vi "Scatter-Gather Read Iterator.vi"(8 "error in (no error)":errorcluster, 9 "Iterations (1000)":i32=110, 10 "Channel Count":i32, 11 "GE 5565PIORC in":refnum<class "GE 5565PIORC.lvclass">) -> (0 "error out":errorcluster, 1 "Histogram Graph":T1(graph), 2 "Metrics":T2 {"Transfer Rate" format="%.2pB/s"; "Duration Std. Dev." format="%.0f µs"; "Duration Average" format="%.0f µs"}, 3 "GE 5565PIORC out":refnum<class "GE 5565PIORC.lvclass">)   [LabVIEW 2016]
uses:
  Source/GE 5565PIORC/GE 5565PIORC.lvclass
  Controls/Throughput Metrics.ctl
  Source/GE 5565PIORC/GE 5565PIORC.lvclass/GE 5565PIORC.ctl
  Source/GE 5565PIORC/VIs/DMA/DMA.Start Transfer.vi
  Source/GE 5565PIORC/VIs/DMA/DMA.Wait for Done Interrupt Event.vi
  Source/GE 5565PIORC/VIs/Interrupts/Discard PXI Interrupt Events.vi
  Source/GE 5565PIORC/VIs/DMA/DMA.Configure.vi
  Source/GE 5565PIORC/VIs/Registers/Local Configuration.DMACSR0.DMA Start.Set.vi
  Source/GE 5565PIORC/VIs/Interrupts/Wait for PXI Interrupt Events.vi
  Source/GE 5565PIORC/VIs/Registers/Local Configuration.DMACSR0.DMA Clear Interrupt.Set.vi
  <vilib>/Utility/error.llb/Clear Errors.vi
  Source/GE 5565PIORC/VIs/Registers/Local Configuration.PCI Address.Set.vi
  Source/GE 5565PIORC/VIs/Registers/Local Configuration.DMADPR0.First Descriptor Address.Set.vi
  Source/GE 5565PIORC/VIs/DMA/DMA.Scatter-Gather.Link Block Descriptors.vi
  Source/GE 5565PIORC/VIs/DMA/DMA.Scatter-Gather.Commit Blocks.vi
  Source/GE 5565PIORC/VIs/Registers/Local Configuration.Local Address.Set.vi
  Source/GE 5565PIORC/VIs/Registers/Local Configuration.Transfer Size.Set.vi
  Source/GE 5565PIORC/VIs/Registers/Local Configuration.DMADPR0.Transfer Direction.Set.vi
  Source/GE 5565PIORC/VIs/Registers/Local Configuration.DMAMODE0.Scatter-Gather Enable.Set.vi
  Source/GE 5565PIORC/VIs/Binary Operations/Set Bits.vi
  Source/GE 5565PIORC/VIs/Binary Operations/Set Bits U32.vi
  Source/GE 5565PIORC/VIs/Registers/Local Configuration.Get Register Offset.vi
  Source/GE 5565PIORC/VIs/Binary Operations/Get Bits.vi
  Source/GE 5565PIORC/VIs/Binary Operations/Get Bits U32.vi
  Source/GE 5565PIORC/VIs/Block Operations/Allocate Multiple Blocks.vi
  Source/GE 5565PIORC/VIs/DMA/DMA.Create Transfer (Multiple Blocks).vi
  Source/GE 5565PIORC/VIs/DMA/DMA.Transfer Size.vi
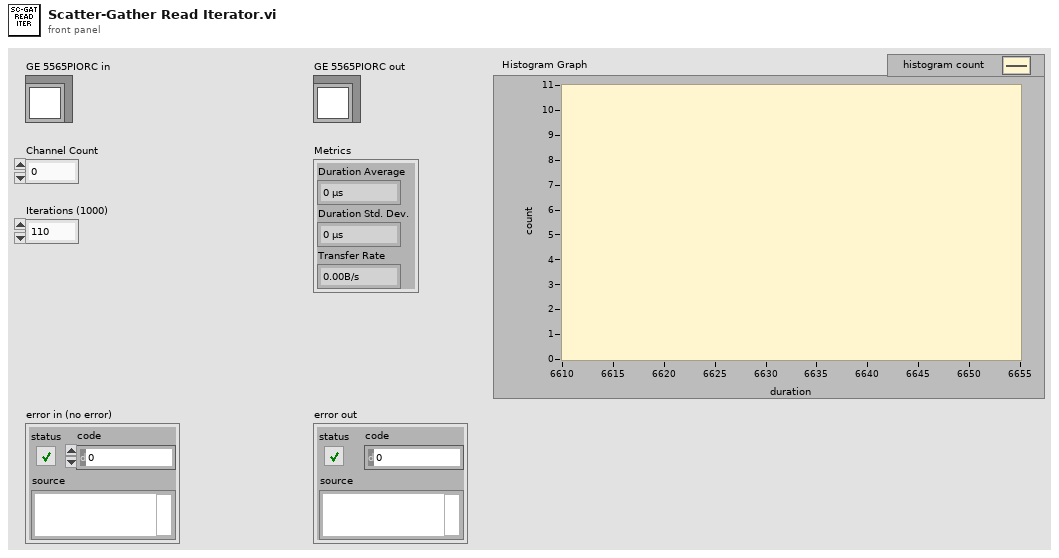
[diagram p1: front panel]
types:
  T1 = cluster{"X Values":dbl[], "Histogram: h(x)":i32[]}
  T2 = typedef "Throughput Metrics.ctl" = cluster{"Duration Average":u32, "Duration Std. Dev.":u32, "Transfer Rate":dbl}
  T3 = typedef "GE 5565PIORC.lvclass/DMA Block Descriptor.ctl" = cluster{"descriptor ptr (VISA)":u32, "descriptor size":u32, "descriptor ptr (aligned)":u32, "data ptr (lower)":u32, "data ptr (upper)":u32, "data size":u32, "next descriptor ptr":u32}
  T4 = typedef "GE 5565PIORC.lvclass/DMA Transfer Spec.ctl" = cluster{"RFM Address":u32, "Block Descriptors":T3[]}
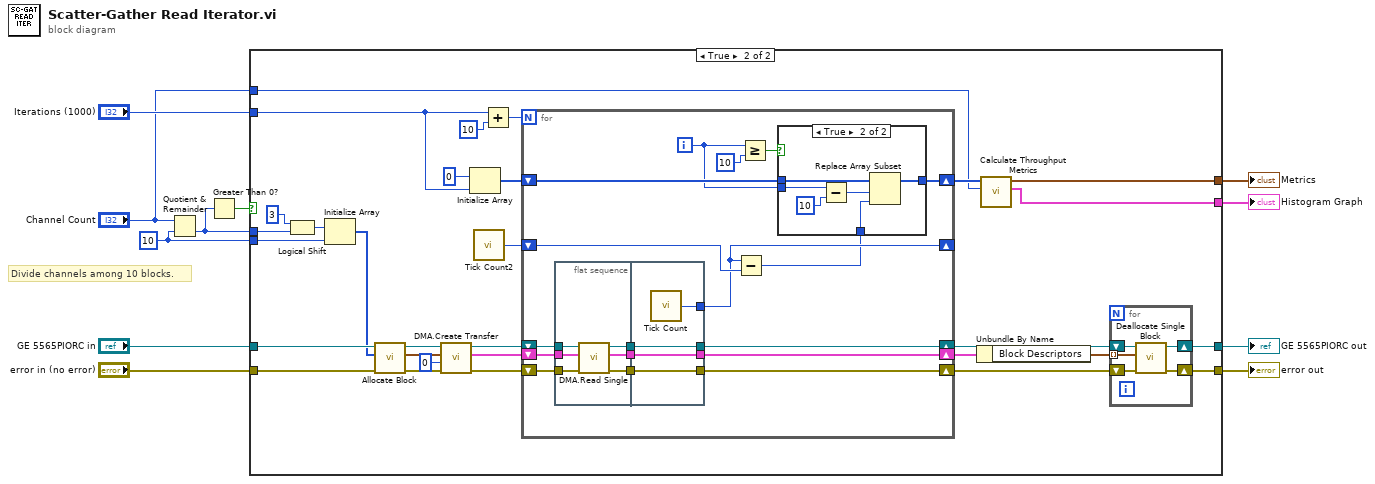
[diagram p0: block diagram]
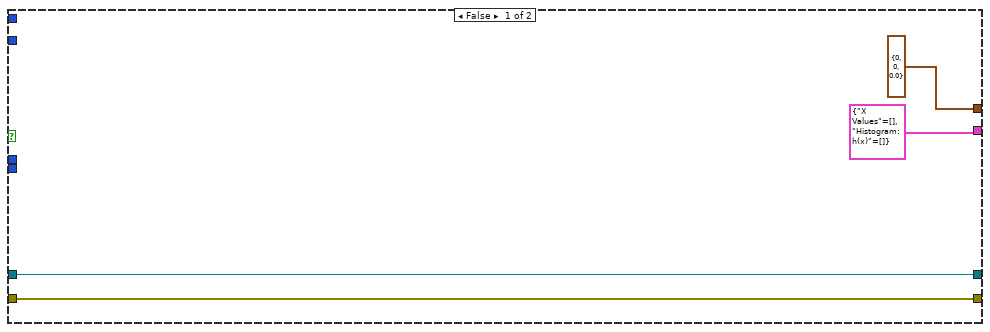
[diagram p2: hidden frame]
diagram:
  w4 = 10 ("y")
  # "Divide channels among 10 blocks."
  n1 = Quotient & Remainder(x="Channel Count", y=w4) -> (floor(x/y)=w2:i32)  [unwired: 1 out]
  n2 = Greater Than 0?(x=w2) -> (x > 0?=w1:bool)
  n3 = case shown="True" w1 {
    tunnel: [w15 w43] -> w11
    tunnel: [w12 w42] -> w10
    tunnel: "Iterations (1000)" -> [_ w36]
    tunnel: [T2 {"Duration Average"=0, "Duration Std. Dev."=0, "Transfer Rate"=0.0} ("Metrics") w32] -> w8
    tunnel: [T1 {"X Values"=[], "Histogram: h(x)"=[]} ("Histogram Graph") w31] -> w7
    tunnel: "GE 5565PIORC in" -> [w12 w27]
    tunnel: "error in (no error)" -> [w15 w26]
    tunnel: w4 -> [_ w22]
    tunnel: w2 -> [_ w21]
    tunnel: "Channel Count" -> [_ w17]
    frame False {
    }
    frame True {
      n4 = Logical Shift(y=i16 3, x=w21) -> (x << y=w20:i32)
      n5 = Initialize Array(w20, w22) -> (w19:i32[])
      n6 = call-poly "Allocate Block.vi"("error in (no error)"=w26, "sizes (bytes)"=w19, "GE 5565PIORC in"=w27) -> ("error out"=w24:errorcluster, "Block Descriptors"=w23:T3[], "GE 5565PIORC out"=w25:refnum<class "GE 5565PIORC.lvclass">)  [unwired: 6 in]
      n7 = call-poly "DMA.Create Transfer.vi"("error in (no error)"=w24, "RFM Offset"=u32 0, "Block Descriptors"=w23, "GE 5565PIORC in"=w25) -> ("error out"=w29:errorcluster, "DMA Transfer Spec"=w28:T4, "GE 5565PIORC out"=w30:refnum<class "GE 5565PIORC.lvclass">)  [unwired: 4 in, 1 out]
      n8 = Initialize Array(u32 0 ("x-y"), w36) -> (w35:u32[])
      n9 = call "Tick Count2"() -> ("Tick Count(uSec)"=w39:u32)
      n10 = Add(x=w36, y=10) -> (x+y=w45:i32)
      n11 = for {
        N: w45 -> [_]
        shift-right: [w58] -> _
        shift-left: w39 -> [w59]
        shift-right: [w61] -> w40
        shift-left: w30 -> [w67]
        shift-right: [w60] -> w41
        shift-left: w29 -> [w66]
        shift-right: [w56] -> w33
        shift-left: w35 -> [w57]
        shift-right: [w51] -> w18
        shift-left: w28 -> [w65]
        i -> [w54]
        n12 = flat-sequence {
          tunnel: w67 -> [w80]
          tunnel: w66 -> [w79]
          tunnel: w65 -> [w78]
          tunnel: [w76] -> w64
          tunnel: [w75] -> w63
          tunnel: [w77] -> w52
          tunnel: [w84] -> w61
          tunnel: w64 -> [w84]
          tunnel: w63 -> [w83]
          tunnel: [w83] -> w60
          tunnel: [w82] -> w58
          tunnel: w52 -> [w81]
          tunnel: [w81] -> w51
          frame #0 {
            n13 = call "DMA.Read Single.vi"("error in (no error)"=w79, "DMA Transfer Spec"=w78, "GE 5565PIORC"=w80) -> ("error out"=w75:errorcluster, "DMA Transfer Spec out"=w77:T4, "GE 5565PIORC out"=w76:refnum<class "GE 5565PIORC.lvclass">)  [unwired: 5 in, 1 out]
          }
          frame #1 {
            n14 = call "Tick Count"() -> ("Tick Count(uSec)"=w82:u32)
          }
        }
        n15 = Subtract(x=w58, y=w59) -> (x-y=w53:u32)
        n16 = Greater Or Equal?(x=w54, y=10) -> (x >= y?=w55:bool)
        n17 = case shown="True" w55 {
          tunnel: w57 -> [w68 w74]
          tunnel: [w68 w73] -> w56
          tunnel: w54 -> [_ w72]
          tunnel: w53 -> [_ w69]
          frame False {
          }
          frame True {
            n18 = Subtract(x=w72, y=10) -> (x-y=w70:i32)
            n19 = Replace Array Subset(array=w74, new element=w69, index=w70) -> (w73:u32[])
          }
        }
      }
      n20 = Unbundle By Name(w18) -> ("Block Descriptors"=w34:T3[])
      n21 = call "Calculate Throughput Metrics.vi"("Channel Count"=w17, "Durations"=w33) -> ("Histogram Graph"=w31:T1, "Metrics"=w32:T2)  [unwired: 8 in]
      n22 = for {
        tunnel: w34 -> [w46] mode=indexing
        shift-right: [w50] -> w43
        shift-left: w41 -> [w48]
        shift-right: [w49] -> w42
        shift-left: w40 -> [w47]
        n23 = call "Deallocate Single Block.vi"("error in (no error)"=w48, "Block Descriptor"=w46, "GE 5565PIORC in"=w47) -> ("error out"=w50:errorcluster, "GE 5565PIORC out"=w49:refnum<class "GE 5565PIORC.lvclass">)  [unwired: 7 in]
      }
    }
  }
  "error out" <- w11
  "GE 5565PIORC out" <- w10
  "Metrics" <- w8
  "Histogram Graph" <- w7
